vi "3DWedgeSet.vi"() -> ()   [LabVIEW 2022 SP3]
panel:
  in  "Geometry":u16(ring)=1 items=["single wedge", "dual wedge", "Outer Rec Hole", "Inner Rect Hole", "single strip", "dual strips", "Cap w/ Rect Cut", "middle pair", "middle w/ circ hole"]
  in  "Case Constant\n(See Context Help)":bool=TRUE
  in  "y span (cm)":i32=2
  in  "freq (MHz)":dbl=4.7 format="%.2f"
  in  "Points":i32=30
  in  "Variables":T1={"sound spd (cm/s)"=150000, "time step (s)"=1e-09} {"time step (s)" format="%.2e"}
  in  "Plane dimensions (cm)":cluster{"x":dbl, "y":dbl, "z":dbl}={"x"=0.2, "y"=0.0, "z"=0.2} {"x" format="%.2f"; "z" format="%.2f"; "y" format="%.2f"}
  in  "Save Options":cluster{"Save image data?":bool, "Path":path}={"Save image data?"=FALSE, "Path"=path "F:/Test"}
  in  "Trans Geometry":cluster{"Radius (cm)":dbl, "h":dbl, "a":dbl}={"Radius (cm)"=9.0, "h"=2.0, "a"=4.0} {"a" format="%.2f"; "h" format="%.2f"; "Radius (cm)" format="%.2f"}
  in  "Number of focal zones":i32=21
  in  "3D Surface":refnum<k7>(container)
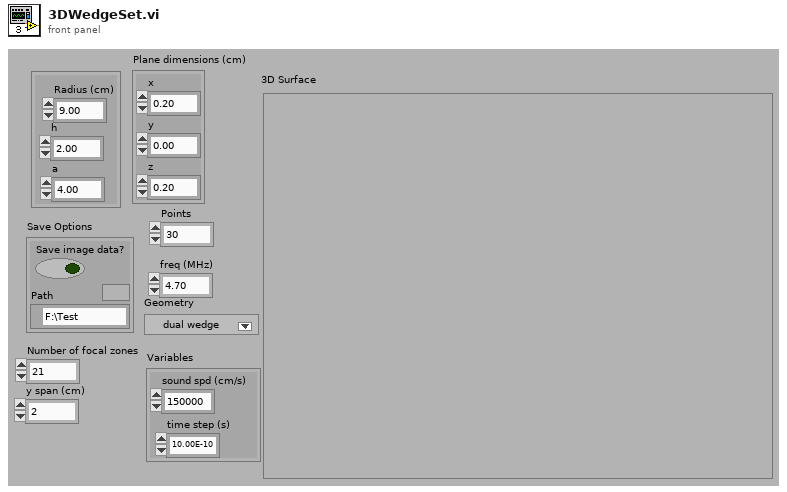
[diagram p1: front panel]
types:
  T1 = cluster{"sound spd (cm/s)":i32, "time step (s)":sgl}
  T2 = typedef "LVRectTypeDef.ctl" = cluster{"left":i16, "top":i16, "right":i16, "bottom":i16}
  T3 = enum16{"open", "open or create", "create or replace", "create"}
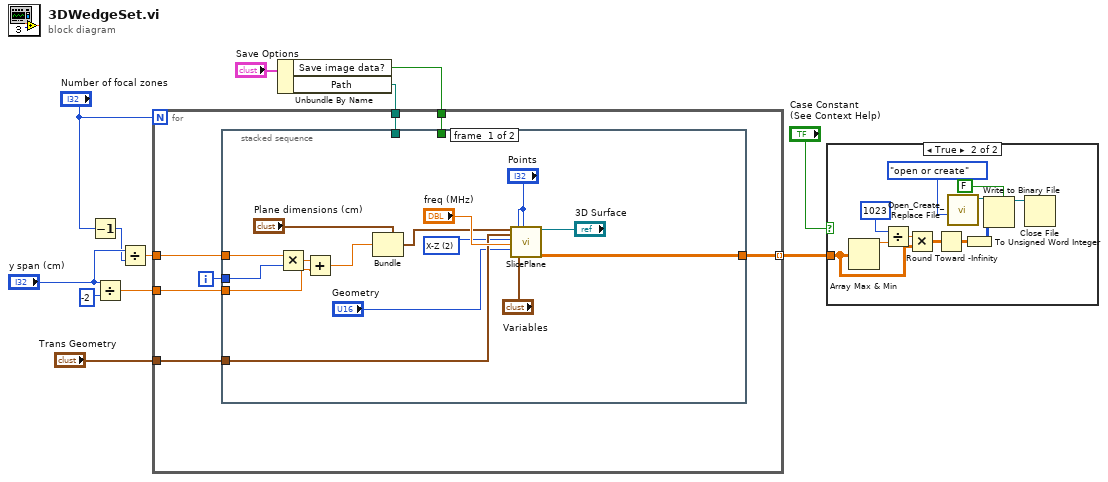
[diagram p0: block diagram]
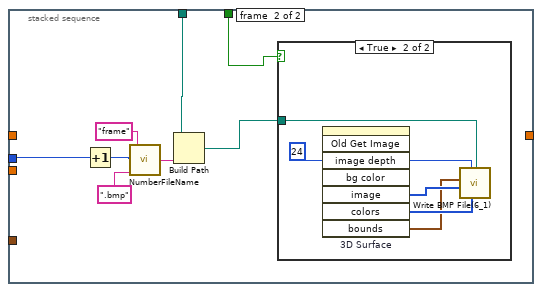
[diagram p3: hidden frame]
diagram:
  n1 = Decrement(x="Number of focal zones") -> (x-1=w1:i32)
  n2 = Divide(x="y span (cm)", y=-2) -> (x/y=w7:dbl)
  n3 = Divide(x="y span (cm)", y=w1) -> (x/y=w12:dbl)
  n4 = Unbundle By Name("Save Options") -> ("Save image data?"=w5:bool, "Path"=w4:path)
  n5 = for {
    N: "Number of focal zones" -> [_]
    tunnel: w12 -> [w19]
    tunnel: "Trans Geometry" -> [w18]
    tunnel: w7 -> [w16]
    tunnel: w5 -> [w15]
    tunnel: w4 -> [w14]
    tunnel: [w13] -> w2 mode=indexing
    i -> [w17]
    n6 = stacked-sequence {
      tunnel: w19 -> [w34 _]
      tunnel: w18 -> [w29 _]
      tunnel: w17 -> [w32 w39]
      tunnel: w16 -> [w25 _]
      tunnel: w15 -> [_ w36]
      tunnel: w14 -> [_ w35]
      tunnel: [w24 _] -> w13
      frame #0 {
        w28 = u16 2 items=["X-Y", "Z-Y", "X-Z"] ("Plane")
        n7 = Multiply(x=w34, y=w32) -> (x*y=w33:dbl)
        n8 = Add(x=w33, y=w25) -> (x+y=w23:dbl)
        n9 = Bundle(cluster="Plane dimensions (cm)", "y"=w23) -> (w20:cluster{"x":dbl, "y":dbl, "z":dbl})  [unwired: 2 in]
        n10 = call "SlicePlane.vi"("Plane dimensions (cm)"=w20, "strip (cm)"=w29, "Plane"=w28, "freq (MHz)"="freq (MHz)", "Geometry"="Geometry", "Points \t1"="Points", "Variables"="Variables", "Points 2"="Points", "3D Surface"="3D Surface") -> ("raw data"=w24:dbl[][])  [unwired: 10 in]
      }
      frame #1 {
        n11 = Increment(x=w39) -> (x+1=w38:i32)
        n12 = call "NumberFileName.vi"("String"=".bmp", "File number"=w38, "file name"="frame") -> ("Numbered File"=w41:string)  [unwired: 1 in]
        n13 = Build Path(base path=w35, name or relative path=w41) -> (appended path=w37:path)
        n14 = case shown="True" w36 {
          tunnel: w37 -> [_ w43]
          frame False {
          }
          frame True {
            w47 = 24
            n15 = invoke on="3D Surface" class="AXCont" method="Old Get Image"("image depth"=w47) -> ("image"=w45:u8[], "colors"=w46:u32[], "bounds"=w44:T2)  [unwired: 7 in, 5 out]
            n16 = call <vilib>:"Write BMP File(6_1).vi"("color table"=w46, "depth"=w47, "flattened image data"=w45, "rect"=w44, "path to BMP file"=w43) -> ()  [unwired: 5 in, 2 out]
          }
        }
      }
    }
  }
  n17 = case shown="True" "Case Constant\n(See Context Help)" {
    tunnel: w2 -> [_ w55]
    frame False {
    }
    frame True {
      n18 = Array Max & Min(array=w55) -> (max value=w57:dbl)  [unwired: 3 out]
      n19 = Divide(x=1023, y=w57) -> (x/y=w56:dbl)
      n20 = Multiply(x=w56, y=w55) -> (x*y=w52:dbl[][][])
      n21 = Round Toward -Infinity(1:w52) -> (0:w50:dbl[][][])
      n22 = call <vilib>:"Open_Create_Replace File.vi"("function (open:0)"=T3."open or create") -> ("refnum"=w54:refnum<file>)  [unwired: 7 in, 3 out]
      n23 = To Unsigned Word Integer(number=w50) -> (unsigned 16bit integer=w49:u16[][][])
      n24 = Write to Binary File(file (use dialog)=w54, data=w49, 5:FALSE ("prepend array or string size? (T)")) -> (refnum out=w53:refnum<file>)  [unwired: 3 in, 2 out]
      n25 = Close File(refnum=w53) -> ()  [unwired: 1 in, 2 out]
    }
  }
